vi "Make Chassis Type Enum.vi"(5 "ProductType":string) -> (2 "ChassisType":T1=enum."C Series 1-Slot")   [LabVIEW 2018, in "Configuration Grandmaster.lvlib" / "Cfg Grandmaster.lvclass"]
uses:
  Cfg Grandmaster.lvclass
  Common/Controls/Chassis Type.ctl
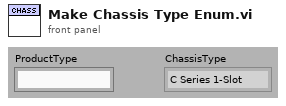
[diagram p1: front panel]
types:
  T1 = typedef "Chassis Type.ctl" = enum16{"Not Supported", "C Series 1-Slot", "C Series 4-Slot", "C Series 8-Slot", "PXI 8-Slot", "PXIe 18-Slot"}
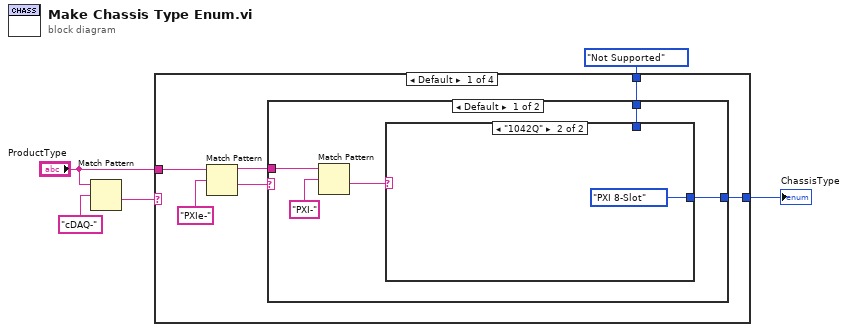
[diagram p0: block diagram]
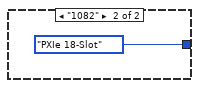
[diagram p3: hidden frame]
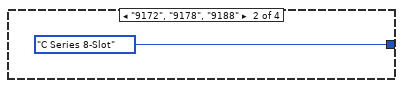
[diagram p4: hidden frame]
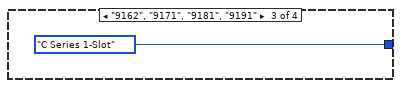
[diagram p5: hidden frame]
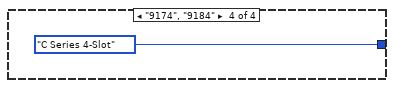
[diagram p6: hidden frame]
diagram:
  n1 = Match Pattern(string="ProductType", regular expression="cDAQ-") -> (after substring=w3:string)  [unwired: 1 in, 3 out]
  n2 = case shown="Default" w3 {
    tunnel: [w11 Chassis_Type."C Series 8-Slot" ("ChassisType") Chassis_Type."C Series 1-Slot" ("ChassisType") Chassis_Type."C Series 4-Slot" ("ChassisType")] -> w5
    tunnel: "ProductType" -> [w10 _ _ _]
    tunnel: Chassis_Type."Not Supported" ("ChassisType") -> [w6 _ _ _]
    frame Default {
      n3 = Match Pattern(string=w10, regular expression="PXIe-") -> (before substring=w7:string, after substring=w8:string)  [unwired: 1 in, 2 out]
      n4 = case shown="Default" w8 {
        tunnel: [w14 Chassis_Type."PXIe 18-Slot" ("ChassisType")] -> w11
        tunnel: w7 -> [w16 _]
        tunnel: w6 -> [w13 _]
        frame Default {
          n5 = Match Pattern(string=w16, regular expression="PXI-") -> (after substring=w12:string)  [unwired: 1 in, 3 out]
          n6 = case shown="\"1042Q\"" w12 {
            tunnel: [w17 Chassis_Type."PXI 8-Slot" ("ChassisType")] -> w14
            tunnel: w13 -> [w17 _]
            frame Default {
            }
            frame "1042Q" {
            }
          }
        }
        frame "1082" {
        }
      }
    }
    frame "9172", "9178", "9188" {
    }
    frame "9162", "9171", "9181", "9191" {
    }
    frame "9174", "9184" {
    }
  }
  "ChassisType" <- w5
